vi "acquire_data_rt.vi"(3 "error in":errorcluster, 5 "Configuration":T1) -> (0 "error out":errorcluster, 1 "timestamp":cluster{"t0":timestamp, "dt":dbl}, 2 "Data":sgl[][](array[numeric]))   [LabVIEW 2013]
uses:
  initialization/configuration.ctl
  initialization/asap_calibration.ctl
  <vilib>/Analysis/Matrix/Datatypes/RealMatrix.ctl
  <vilib>/DAQmx/read.llb/DAQmx Read (Analog 2D DBL NChan NSamp).vi
  <vilib>/DAQmx/miscellaneous.llb/DAQmx Fill In Error Info.vi
  <resource>/objmgr/daqmx.rc
  <vilib>/Analysis/Matrix/NI_Matrix.lvlib
panel:
  out "Synch iterations":i32
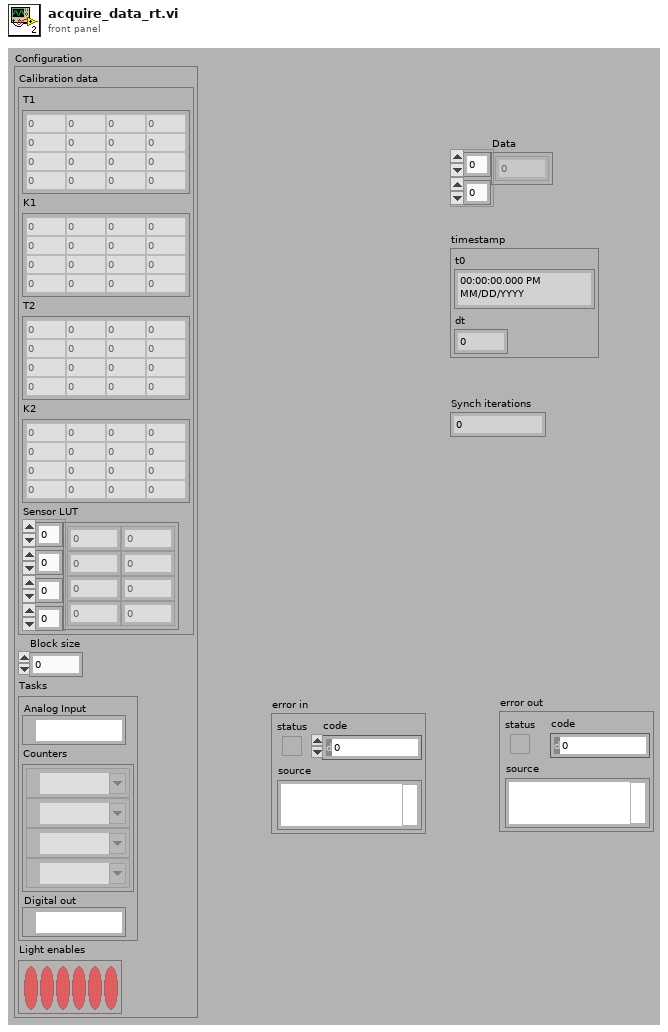
[diagram p1: front panel]
types:
  T1 = typedef "configuration.ctl" = cluster{"Calibration data":T2, "Block size":i32, "Tasks":cluster{"Analog Input":refnum<k21>, "Counters":refnum<k21>[], "Digital out":refnum<k21>}, "Light enables":bool[]}
  T2 = typedef "asap_calibration.ctl" = cluster{"T1":T3, "K1":T3, "T2":T3, "K2":T3, "Sensor LUT":sgl[][][][]}
  T3 = typedef "NI_Matrix.lvlib/RealMatrix.ctl" = dbl[][]
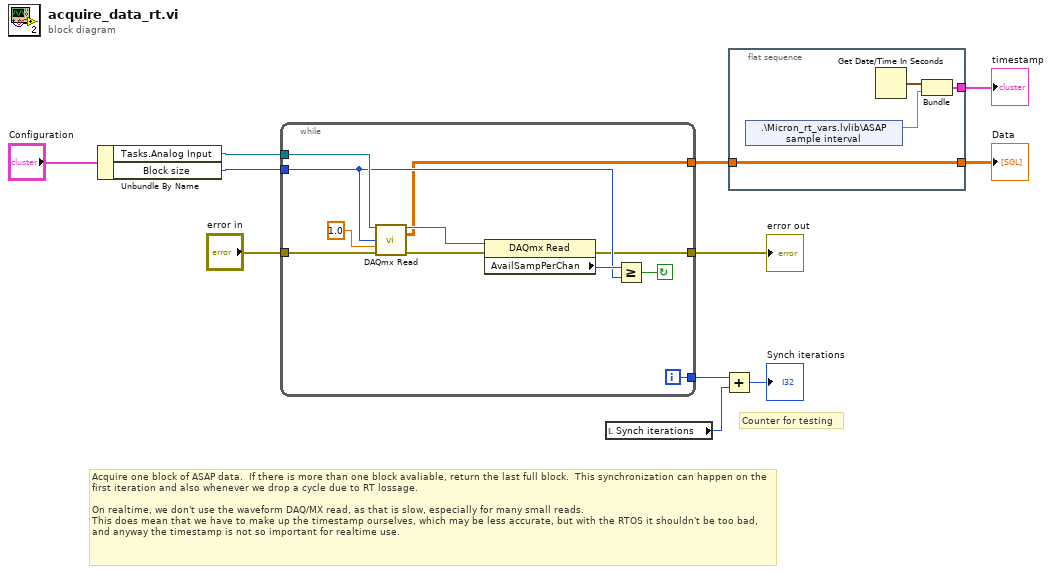
[diagram p0: block diagram]
diagram:
  # "Counter for testing"
  # "Acquire one block of ASAP data.  If there is more than one block avaliable, return the last full block.  This synchronization can happen on the first iteration and also whenever we drop a cycle due to RT lossage.\n\nOn realtime, we don't use the waveform DAQ/MX read, as that is slow, especially for many small reads.\nThis does mean that we have to make up the timestamp ourselves, which may be less accurate, but with the RTOS it shouldn't be too bad, and anyway the timestamp is not so important for realtime use."
  n1 = Unbundle By Name("Configuration") -> ("Tasks.Analog Input"=w10:refnum<k21>, "Block size"=w9:i32)
  n2 = while {
    tunnel: w10 -> [w22]
    tunnel: "error in" -> [w21]
    tunnel: [w15] -> w7
    tunnel: w9 -> [w16]
    tunnel: [w14] -> w3
    tunnel: [w13] -> w6
    i -> [w13]
    stop <- w18 continue-if-true
    n3 = call-poly <vilib>:"DAQmx Read.vi"("task/channels in"=w22, "number of samples per channel"=w16, "timeout"=1.0, "error in"=w21) -> ("task out"=w19:refnum<k21>, "data"=w14:dbl[][], "error out"=w12:errorcluster)  [unwired: 9 out]
    n4 = property class="DAQmx Read"(reference=w19, error in=w12) -> (error out=w15:errorcluster, "AvailSampPerChan"=w17:u32)  [unwired: 1 out]
    n5 = Greater Or Equal?(x=w17, y=w16) -> (x >= y?=w18:bool)
  }
  "error out" <- w7
  n6 = local read "Synch iterations"() -> (w4:i32)
  n7 = Add(x=w6, y=w4) -> (x+y=→"Synch iterations":i32)
  n8 = flat-sequence {
    tunnel: w3 -> [w25]
    tunnel: [w25] -> w2
    tunnel: [w24] -> w1
    frame #0 {
      n9 = shared-variable ".\\Micron_rt_vars.lvlib\\ASAP sample interval"() -> (w23:dbl)  [unwired: 2 out]
      n10 = Get Date/Time In Seconds() -> (seconds since 1Jan1904=w26:timestamp)
      n11 = Bundle("seconds since 1Jan1904"=w26, w23) -> (w24:cluster{"seconds since 1Jan1904":timestamp, dbl})  [unwired: 1 out]
    }
  }
  "Data" <- w2
  "timestamp" <- w1
